vi "SDO_DRIVE_MODULE_ACT.vi"(6 "Pass_Through_Time":dbl=-1.0 format="%33.4f", 8 "AllSwervePosInDeadband":bool=TRUE, 9 "Swerve State":T1={"Speed"=0.0, "Angle"={"VALUE"=0.0, "COS"=1.0, "SIN"=0.0}} {"Angle"."SIN" format="%13.4f"; "Angle"."COS" format="%13.4f"; "Angle"."VALUE" format="%13.4f"}, 10 "Swerve Dmd":T1={"Speed"=0.0, "Angle"={"VALUE"=0.0, "COS"=1.0, "SIN"=0.0}} {"Angle"."SIN" format="%13.4f"; "Angle"."COS" format="%13.4f"; "Angle"."VALUE" format="%13.4f"}, 11 "Swerve Module TypDef":T3) -> (0 "SwerveOnTarget":bool, 1 "SwervePosError":dbl, 2 "Swerve Motor Dmd":dbl, 3 "Wheel Motor Dmd":dbl, 4 "WheelSpeedErr":dbl, 5 "Optimized Swerve \nDmd Radians":dbl, 7 "Optimized Speed \nDmd M/S":dbl)   [LabVIEW 2019]
uses:
  PPS_DRIVE_MODULE_TYPDEF.ctl
  <vilib>/Rock Robotics/WPI/MotorControl/WPI_MotorControlDeviceRef.ctl
  <vilib>/Rock Robotics/WPI/MotorControl/WPI_MotorControlType.ctl
  <vilib>/Rock Robotics/SystemInterfaces/DIO/FPGA_DIOPWMChannel.ctl
  <vilib>/Rock Robotics/WPI/PWM/WPI_PWMDeadband.ctl
  <vilib>/Rock Robotics/SystemInterfaces/DIO/FPGA_DIOChannel.ctl
  <vilib>/Rock Robotics/WPI/Encoder/WPI_EncoderDevRef.ctl
  <vilib>/Rock Robotics/SystemInterfaces/Encoder/FPGA_EncoderIdx.ctl
  <vilib>/Rock Robotics/SystemInterfaces/Counter/FPGA_CounterCtrSystemIndex.ctl
  <vilib>/Rock Robotics/WPI/Encoder/WPI_EncoderType.ctl
  <vilib>/Rock Robotics/WPI/ThirdParty/JAS_Junk/TrajLib/TypeDef/SWERVE_DRIVE_MODULE_STATE.ctl
  <vilib>/Rock Robotics/WPI/ThirdParty/JAS_Junk/TrajLib/TypeDef/ROTATION2D.ctl
  <vilib>/Rock Robotics/WPI/ThirdParty/JAS_Junk/TrajLib/TypeDef/X_Y_PAIR.ctl
  <vilib>/Rock Robotics/WPI/ThirdParty/JAS_Junk/TrajLib/VI/Util_GetTime_U32.vi
  <vilib>/Rock Robotics/WPI/ThirdParty/JAS_Junk/TrajLib/Rotation2d_Minus.vi
  <vilib>/Rock Robotics/WPI/ThirdParty/JAS_Junk/TrajLib/Rotation2d_GetRadians.vi
  <vilib>/Rock Robotics/WPI/ThirdParty/JAS_Junk/TrajLib/SwerveModuleState_New.vi
  <vilib>/Rock Robotics/WPI/ThirdParty/JAS_Junk/TrajLib/Rotation2d_RotateBy.vi
  <vilib>/Rock Robotics/WPI/ThirdParty/JAS_Junk/TrajLib/Rotation2d_CreateAngle.vi
  <vilib>/Rock Robotics/WPI/ThirdParty/JAS_Junk/TrajLib/ProfiledPIDController_SetPID.vi
  <vilib>/Rock Robotics/WPI/ThirdParty/JAS_Junk/TrajLib/ProfiledPIDController_SetIntegratorRange.vi
  <vilib>/Rock Robotics/WPI/ThirdParty/JAS_Junk/TrajLib/ProfiledPIDController_SetTolerance_PosVel.vi
  <vilib>/Rock Robotics/WPI/ThirdParty/JAS_Junk/TrajLib/ProfiledPIDController_DisableContInput.vi
  <vilib>/Rock Robotics/WPI/ThirdParty/JAS_Junk/TrajLib/ProfiledPIDController_EnableContInput.vi
  <vilib>/Rock Robotics/WPI/ThirdParty/JAS_Junk/TrajLib/ProfiledPIDController_Reset_PosOnly.vi
  <vilib>/Rock Robotics/WPI/ThirdParty/JAS_Junk/TrajLib/ProfiledPIDController_NewPeriod.vi
  <vilib>/Rock Robotics/WPI/ThirdParty/JAS_Junk/TrajLib/ProfiledPIDController_Calculate_Meas_Goal.vi
  <vilib>/Rock Robotics/WPI/ThirdParty/JAS_Junk/TrajLib/ProfiledPIDController_AtGoal.vi
  <vilib>/Rock Robotics/WPI/ThirdParty/JAS_Junk/TrajLib/ProfiledPIDController_AtSetpoint.vi
  <vilib>/Rock Robotics/WPI/ThirdParty/JAS_Junk/TrajLib/ProfiledPIDController_SetConstraints.vi
  <vilib>/Rock Robotics/WPI/ThirdParty/JAS_Junk/TrajLib/VI/FunctionGenerator_New.vi
  <vilib>/Rock Robotics/WPI/ThirdParty/JAS_Junk/TrajLib/VI/FunctionGenerator_Calculate.vi
  <vilib>/Rock Robotics/WPI/ThirdParty/JAS_Junk/TrajLib/PIDController_AtSetpoint.vi
  <vilib>/Rock Robotics/WPI/ThirdParty/JAS_Junk/TrajLib/PIDController_SetPIDF.vi
  <vilib>/Rock Robotics/WPI/ThirdParty/JAS_Junk/TrajLib/PIDController_SetDerivativeFilter.vi
  <vilib>/Rock Robotics/WPI/ThirdParty/JAS_Junk/TrajLib/PIDController_SetIntegratorRange.vi
  <vilib>/Rock Robotics/WPI/ThirdParty/JAS_Junk/TrajLib/PIDController_SetTolerancePandV.vi
  <vilib>/Rock Robotics/WPI/ThirdParty/JAS_Junk/TrajLib/PIDController_DisableContinousInput.vi
  <vilib>/Rock Robotics/WPI/ThirdParty/JAS_Junk/TrajLib/PIDController_EnableContinousInput.vi
  <vilib>/Rock Robotics/WPI/ThirdParty/JAS_Junk/TrajLib/PIDController_Reset.vi
  <vilib>/Rock Robotics/WPI/ThirdParty/JAS_Junk/TrajLib/PIDController_New.vi
  <vilib>/Rock Robotics/WPI/ThirdParty/JAS_Junk/TrajLib/PIDController_SetOutputLimits.vi
  <vilib>/Rock Robotics/WPI/ThirdParty/JAS_Junk/TrajLib/SlewRateLimiter_New.vi
  <vilib>/Rock Robotics/WPI/ThirdParty/JAS_Junk/TrajLib/SlewRateLimiter_Reset.vi
  <vilib>/Rock Robotics/WPI/ThirdParty/JAS_Junk/TrajLib/SlewRateLimiter_Calculate.vi
  <vilib>/Rock Robotics/WPI/ThirdParty/JAS_Junk/TrajLib/SlewRateLimiter_SetRate.vi
  <vilib>/Rock Robotics/WPI/ThirdParty/JAS_Junk/TrajLib/Rotation2d_UnaryMinus.vi
  <vilib>/Rock Robotics/WPI/ThirdParty/JAS_Junk/TrajLib/Rotation2d_CreateXY.vi
  <vilib>/Rock Robotics/WPI/ThirdParty/JAS_Junk/TrajLib/PIDController_SetPID.vi
  <vilib>/Rock Robotics/WPI/ThirdParty/JAS_Junk/TrajLib/TrapProfState_New.vi
  <vilib>/Rock Robotics/WPI/ThirdParty/JAS_Junk/TrajLib/ProfiledPIDController_Reset.vi
  <vilib>/Rock Robotics/WPI/ThirdParty/JAS_Junk/TrajLib/PIDController_NewPeriod.vi
  <vilib>/Rock Robotics/SystemInterfaces/NetworkCommunication/NetComm_UsageReport_report.vi
  <vilib>/Rock Robotics/WPI/ThirdParty/JAS_Junk/TrajLib/ProfiledPIDController_SetGoal_PosOnly.vi
  <vilib>/Rock Robotics/WPI/ThirdParty/JAS_Junk/TrajLib/ProfiledPIDController_Calculate_Meas.vi
  <vilib>/Rock Robotics/WPI/ThirdParty/JAS_Junk/TrajLib/TrapProfState_Equals.vi
  <vilib>/Rock Robotics/WPI/ThirdParty/JAS_Junk/TrajLib/Util_CalcDist.vi
  <vilib>/Rock Robotics/WPI/ThirdParty/JAS_Junk/TrajLib/ProfiledPIDController_SetGoal.vi
  <vilib>/Rock Robotics/WPI/ThirdParty/JAS_Junk/TrajLib/PIDController_Calculate_SP_PV.vi
  <vilib>/Rock Robotics/WPI/ThirdParty/JAS_Junk/TrajLib/TrapProfile_New.vi
  <vilib>/Rock Robotics/WPI/ThirdParty/JAS_Junk/TrajLib/ProfiledPIDController_GetPeriod.vi
  <vilib>/Rock Robotics/WPI/ThirdParty/JAS_Junk/TrajLib/TrapProfile_Calculate.vi
  <vilib>/Rock Robotics/WPI/ThirdParty/JAS_Junk/TrajLib/ControllerUtil_GetModulusError.vi
  <vilib>/Rock Robotics/WPI/ThirdParty/JAS_Junk/TrajLib/PIDController_SetSetpoint.vi
  <vilib>/Rock Robotics/WPI/ThirdParty/JAS_Junk/TrajLib/PIDController_Calculate_PV.vi
  <vilib>/Rock Robotics/WPI/ThirdParty/JAS_Junk/TrajLib/TrapProfile_ShouldFlipAcceleration.vi
  <vilib>/Rock Robotics/WPI/ThirdParty/JAS_Junk/TrajLib/TrapProfile_Direct.vi
  <vilib>/Rock Robotics/WPI/ThirdParty/JAS_Junk/TrajLib/PIDController_GetPeriod.vi
  <vilib>/Rock Robotics/WPI/ThirdParty/JAS_Junk/TrajLib/VI/Util_GetTime_U64.vi
  <vilib>/gmath/interp.llb/Search Ordered Table.vi
  <vilib>/Rock Robotics/WPI/ThirdParty/JAS_Junk/TrajLib/Globals/Util_LibraryGlobals.vi
  SDO_DRIVE_GLOBALS.vi
  <vilib>/Rock Robotics/WPI/ThirdParty/JAS_Junk/TrajLib/PIDController_AdvCalculate_FF_Sp_Pv.vi
  <vilib>/Rock Robotics/WPI/ThirdParty/JAS_Junk/TrajLib/Trajectory_Library.lvlib
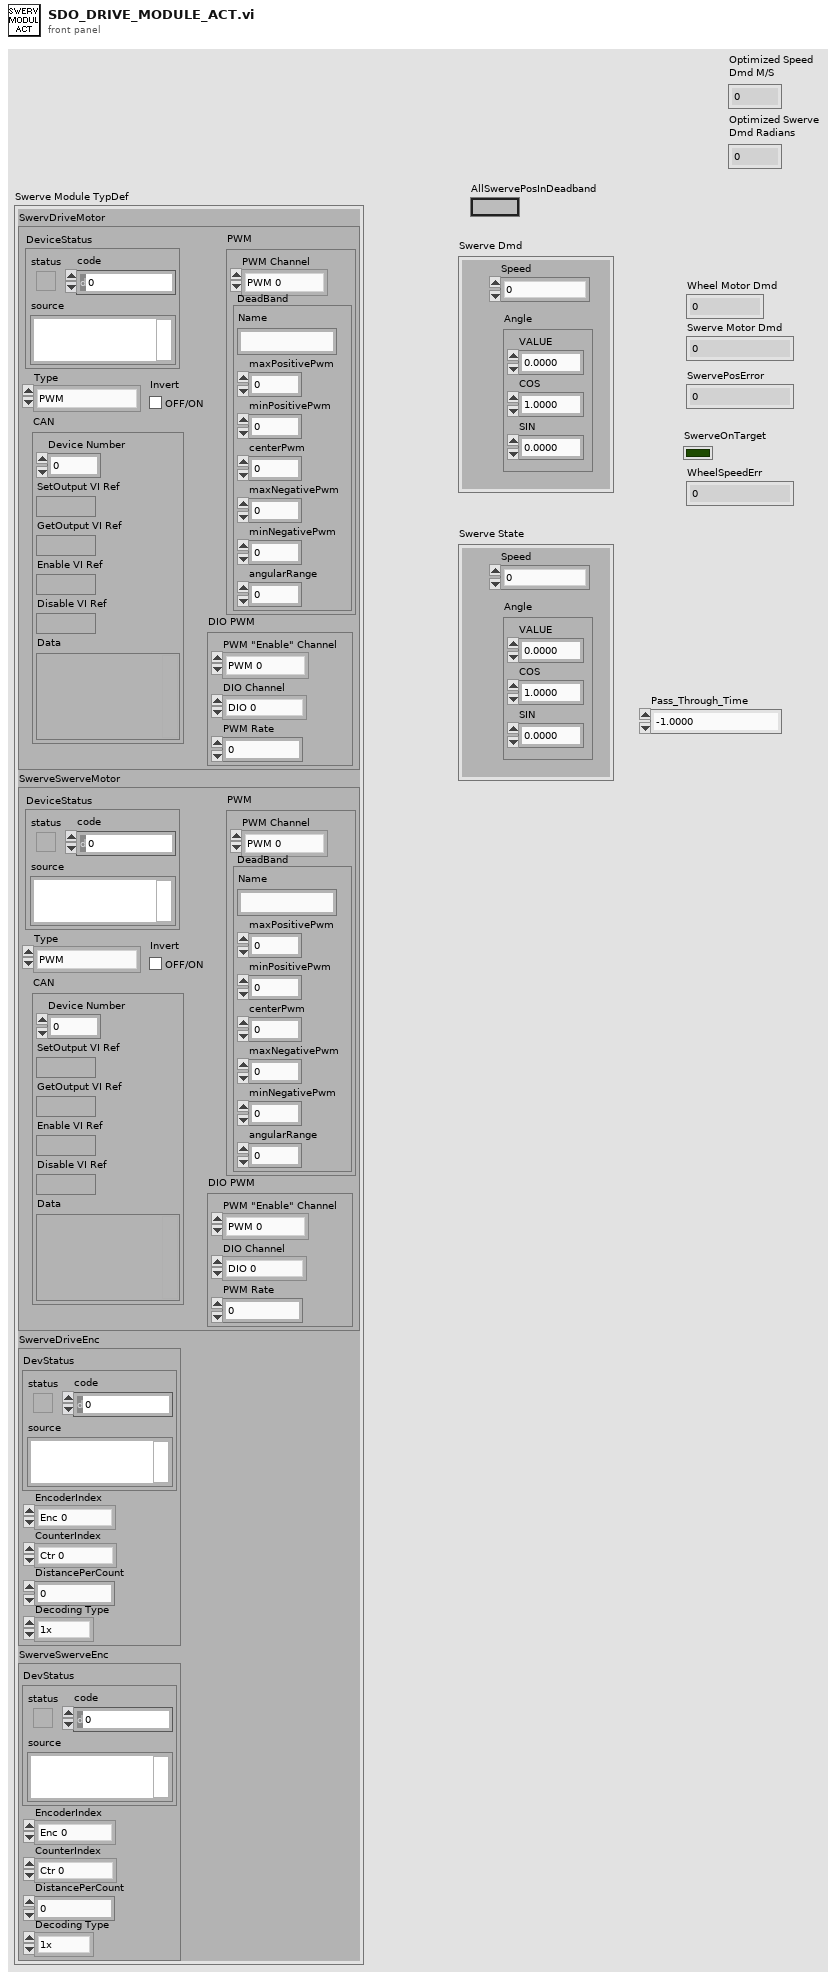
[diagram p1: front panel]
types:
  T1 = typedef "Trajectory_Library.lvlib/SWERVE_DRIVE_MODULE_STATE.ctl" = cluster{"Speed":dbl, "Angle":T2}
  T2 = typedef "Trajectory_Library.lvlib/ROTATION2D.ctl" = cluster{"VALUE":dbl, "COS":dbl, "SIN":dbl}
  T3 = typedef "PPS_DRIVE_MODULE_TYPDEF.ctl" = cluster{"SwervDriveMotor":T4, "SwerveSwerveMotor":T4, "SwerveDriveEnc":T9, "SwerveSwerveEnc":T9}
  T4 = typedef "WPI_MotorControlDeviceRef.ctl" = cluster{"DeviceStatus":errorcluster, "Type":T5, "PWM":cluster{"PWM Channel":T6, "DeadBand":T7}, "CAN":cluster{"Device Number":u8, "SetOutput VI Ref":variant, "GetOutput VI Ref":variant, "Enable VI Ref":variant, "Disable VI Ref":variant, "Data":variant}, "Invert":bool, "DIO PWM":cluster{"PWM \"Enable\" Channel":T6, "DIOChannel":T8, "PWM Rate":dbl}}
  T5 = typedef "WPI_MotorControlType.ctl" = enum16{"PWM", "CAN", "DIO PWM"}
  T6 = typedef "FPGA_DIOPWMChannel.ctl" = enum8{"PWM 0", "PWM 1", "PWM 2", "PWM 3", "PWM 4", "PWM 5", "PWM 6", "PWM 7", "PWM 8", "PWM 9", "PWM MXP 0", "PWM MXP 1", "PWM MXP 2", "PWM MXP 3", "PWM MXP 4", "PWM MXP 5", "PWM MXP 6", "PWM MXP 7", "PWM MXP 8", "PWM MXP 9", "Invalid"}
  T7 = typedef "WPI_PWMDeadband.ctl" = cluster{"Name":string, "maxPositivePwm":i32, "minPositivePwm":i32, "centerPwm":i32, "maxNegativePwm":i32, "minNegativePwm":i32, "angularRange":u16}
  T8 = typedef "FPGA_DIOChannel.ctl" = enum8{"DIO 0", "DIO 1", "DIO 2", "DIO 3", "DIO 4", "DIO 5", "DIO 6", "DIO 7", "DIO 8", "DIO 9", "DIO MXP 0", "DIO MXP 1", "DIO MXP 2", "DIO MXP 3", "DIO MXP 4", "DIO MXP 5", "DIO MXP 6", "DIO MXP 7", "DIO MXP 8", "DIO MXP 9", "DIO MXP 10", "DIO MXP 11", "DIO MXP 12", "DIO MXP 13", "DIO MXP 14", "DIO MXP 15", "SPI Port CS1", "SPI Port CS2", "SPI Port CS3", "SPI Port MISO", "SPI Port MOSI", "Invalid"}
  T9 = typedef "WPI_EncoderDevRef.ctl" = cluster{"DevStatus":errorcluster, "EncoderIndex":T10, "CounterIndex":T11, "DistancePerCount":dbl, "Decoding Type":T12}
  T10 = typedef "FPGA_EncoderIdx.ctl" = enum8{"Enc 0", "Enc 1", "Enc 2", "Enc 3", "Enc 4", "Enc 5", "Enc 6", "Enc 7", "Invalid"}
  T11 = typedef "FPGA_CounterCtrSystemIndex.ctl" = enum8{"Ctr 0", "Ctr 1", "Ctr 2", "Ctr 3", "Ctr 4", "Ctr 5", "Ctr 6", "Ctr 7", "Invalid"}
  T12 = typedef "WPI_EncoderType.ctl" = enum16{"1x", "2x", "4x"}
  T13 = typedef "Trajectory_Library.lvlib/X_Y_PAIR.ctl" = cluster{"X":dbl, "Y":dbl}
  T14 = typedef "Trajectory_Library.lvlib/PID_TUNING.ctl" = cluster{"Kp":dbl, "Ki":dbl, "Kd":dbl, "MaximumIntegral":dbl, "MinimumIntegral":dbl}
  T15 = typedef "Trajectory_Library.lvlib/PID_ERROR_TOLERANCE.ctl" = cluster{"PositionTolerance":dbl, "VelocityTolerance":dbl}
  T16 = typedef "Trajectory_Library.lvlib/PID_INPUT_LIMITS.ctl" = cluster{"MaxInput":dbl, "MinInput":dbl, "Continuous":bool}
  T17 = typedef "Trajectory_Library.lvlib/TRAPEZOID_PROFILE_CONSTRAINT.ctl" = cluster{"MaxVelocity":dbl, "MaxAcceleration":dbl}
  T18 = typedef "Trajectory_Library.lvlib/PosCtrl_Tuning_Type.ctl" = cluster{"Slope":dbl, "Offset":dbl, "Error Deadband":dbl, "At Reference Count":i32, "Negate Output":bool, "Max Allowd Position":dbl, "Min Allowd Position":dbl}
  T19 = typedef "Trajectory_Library.lvlib/PID_ADV_LIMITS.ctl" = cluster{"MaxInput":dbl, "MinInput":dbl, "Continuous":bool, "MaxOutput":dbl, "MinOutput":dbl}
  T20 = typedef "Trajectory_Library.lvlib/PID_ADV_TUNING.ctl" = cluster{"Kf":dbl, "Kp":dbl, "Ki":dbl, "Kd":dbl, "MaximumIntegral":dbl, "MinimumIntegral":dbl, "Filter Derivative":bool}
  T21 = typedef "Trajectory_Library.lvlib/PID_CONTROLLER.ctl" = cluster{"Kp":dbl, "Ki":dbl, "Kd":dbl, "Period":dbl, "Max_Integral":dbl, "Min_Integral":dbl, "Max_Input":dbl, "Min_Input":dbl, "Continuous":bool, "PositionError":dbl, "VelocityError":dbl, "PrevError":dbl, "TotalError":dbl, "PositionTolerance":dbl, "VelocityTolerance":dbl, "SetPoint":dbl, "Kf":dbl, "Prev_Deriv":dbl, "Prev_Deriv 2":dbl, "DerivativeFilter":bool, "Min_Output":dbl, "Max_Output":dbl, "Prev_F_P":dbl, "Prev_F_P_2":dbl, "AntiWindupActive":bool, "Measurement":dbl}
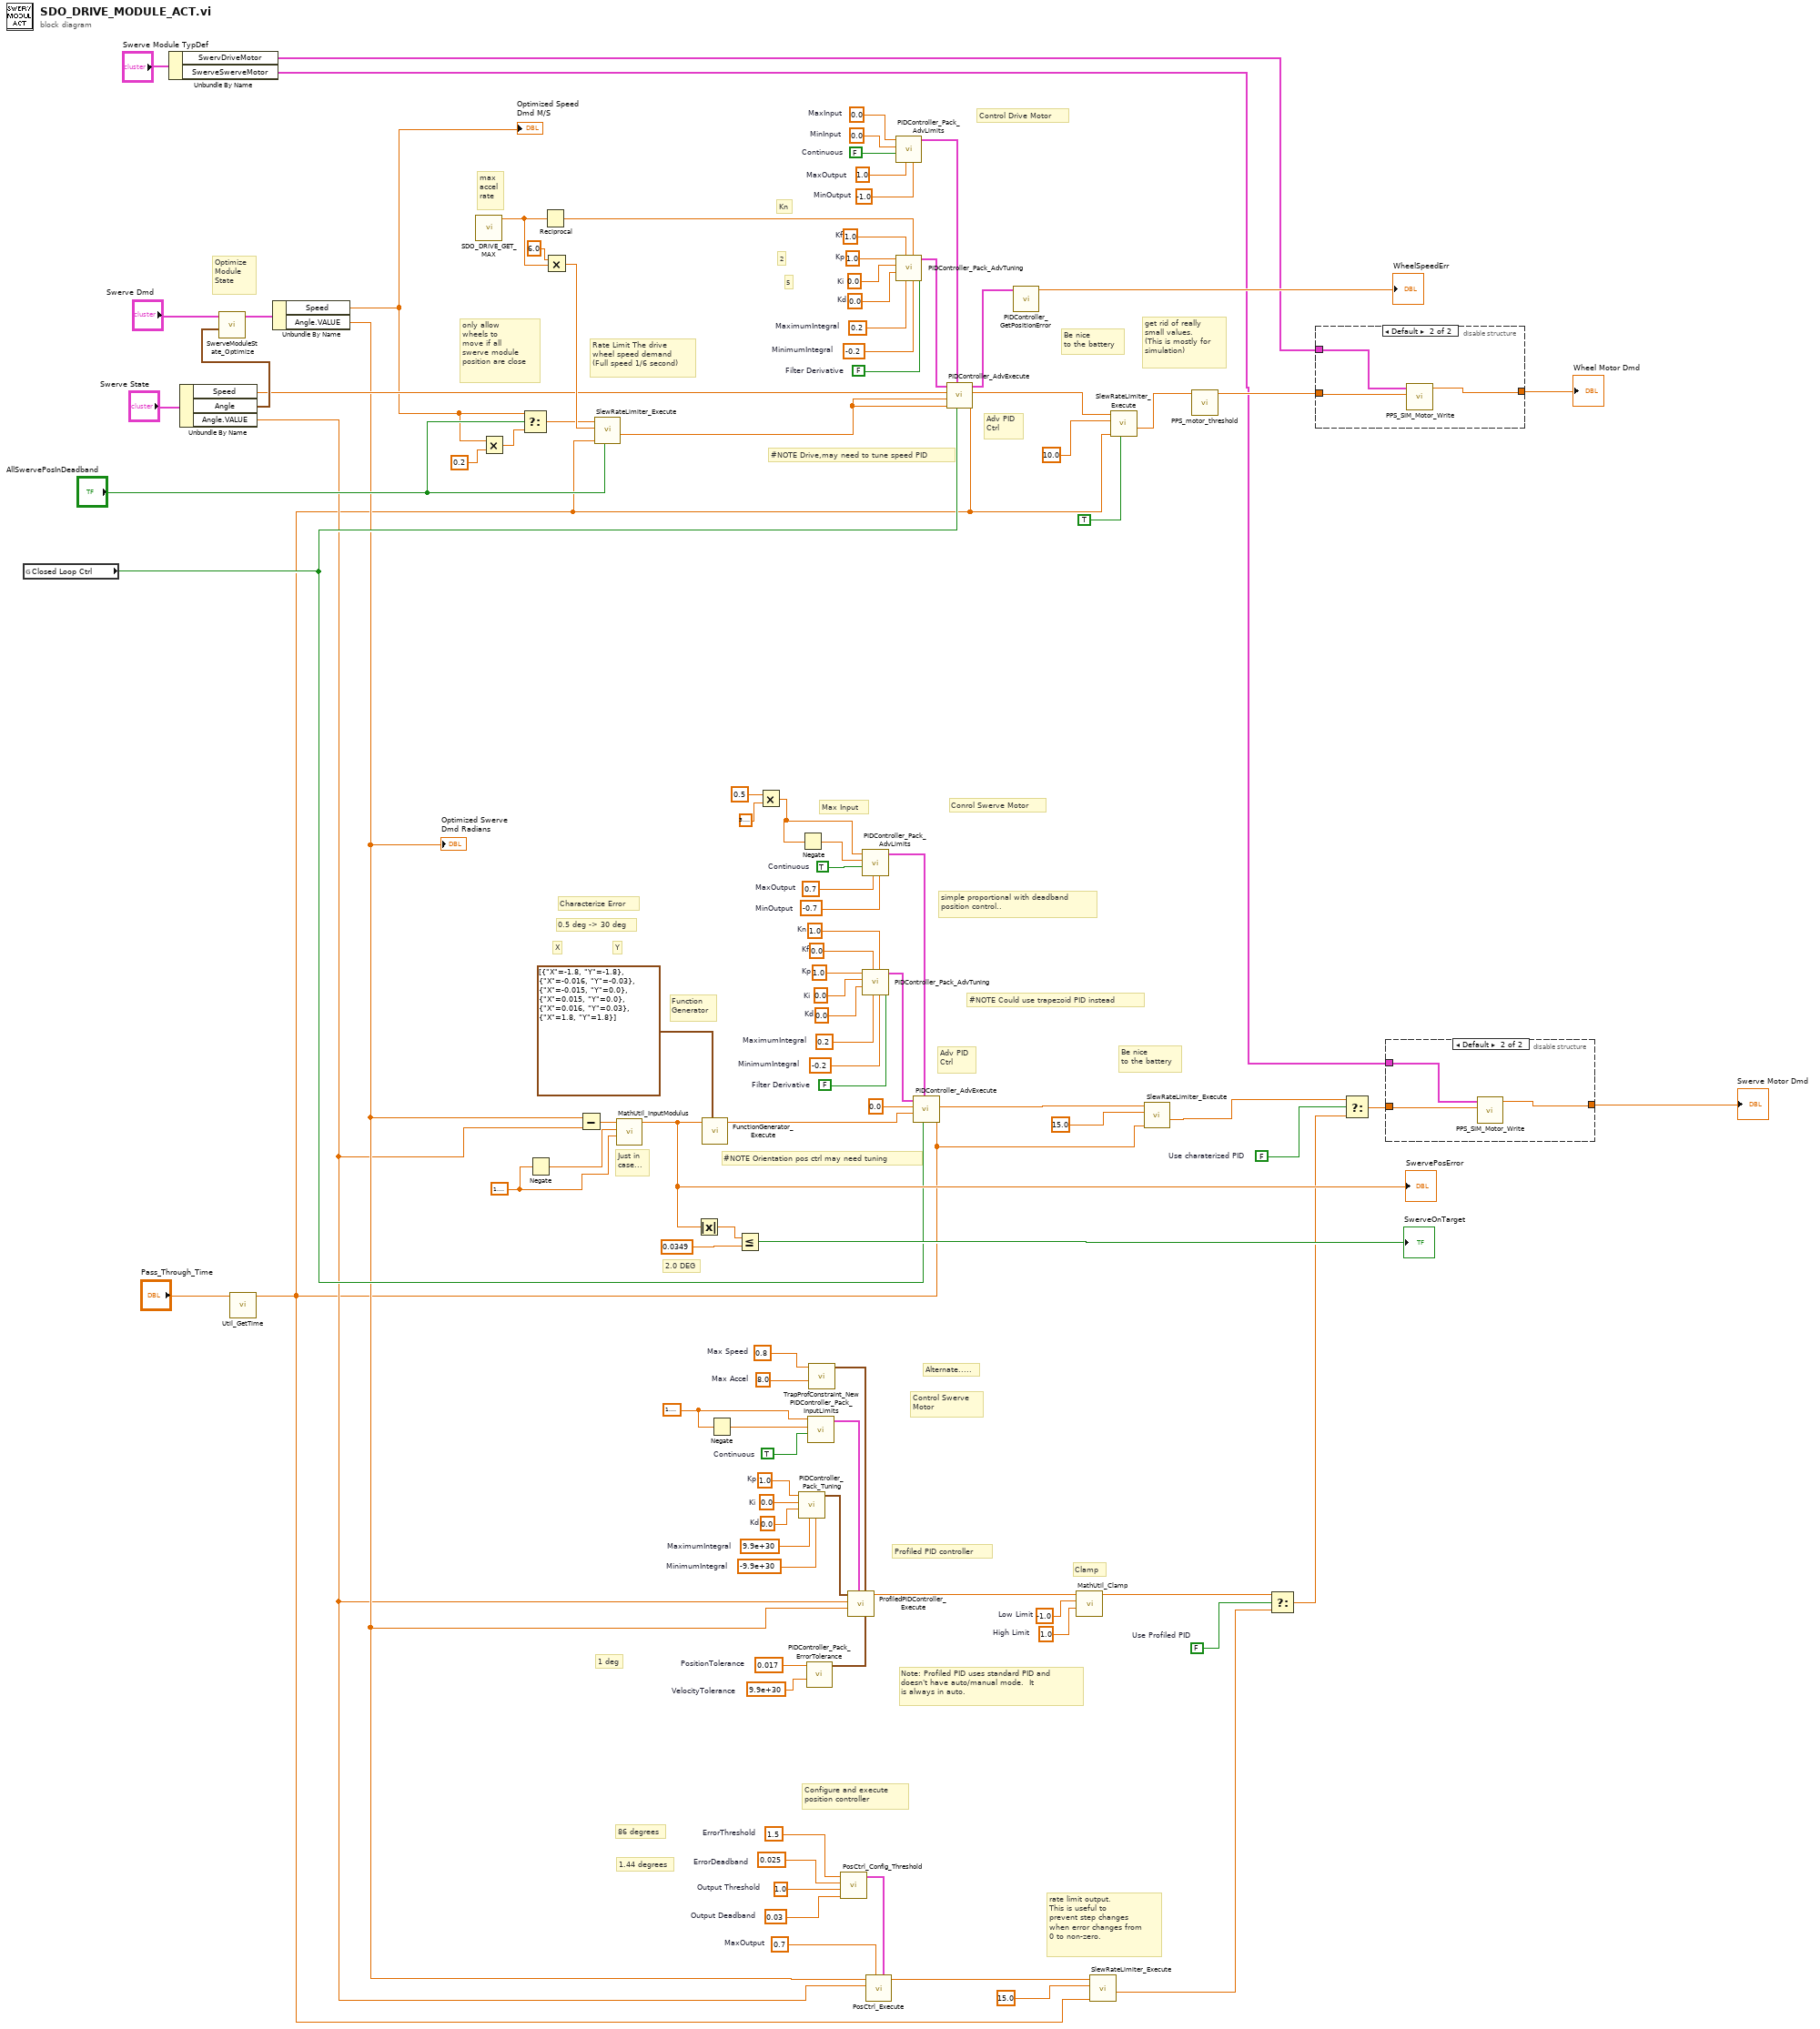
[diagram p0: block diagram]
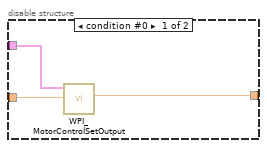
[diagram p2: hidden frame]
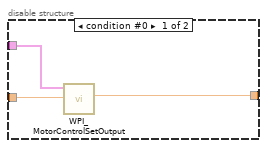
[diagram p3: hidden frame]
diagram:
  w3 = FALSE  # Use charaterized PID
  w11 = FALSE  # Use Profiled PID
  w18 = 0.7  # MaxOutput
  w16 = 1.5  # ErrorThreshold
  w15 = 0.025  # ErrorDeadband
  w14 = 1.0  # Output Threshold
  w13 = 0.03  # Output Deadband
  w22 = 1.5707963267948966
  w23 = 1.5707963267948966
  w29 = 1.0  # High Limit
  w28 = -1.0  # Low Limit
  w54 = 0.017  # PositionTolerance
  w53 = 9.9e+30  # VelocityTolerance
  w51 = 0.8  # Max Speed
  w50 = 8.0  # Max Accel
  w48 = TRUE  # Continuous
  w47 = 1.0  # Kp
  w46 = 0.0  # Ki
  w45 = 0.0  # Kd
  w44 = 9.9e+30  # MaximumIntegral
  w43 = -9.9e+30  # MinimumIntegral
  w78 = 1.0  # Kp
  w77 = 0.0  # Ki
  w76 = 0.0  # Kd
  w75 = 1.0  # Kf
  w74 = 0.2  # MaximumIntegral
  w73 = -0.2  # MinimumIntegral
  w72 = FALSE  # Filter Derivative
  w70 = 0.0  # MinInput
  w69 = FALSE  # Continuous
  w68 = 1.0  # MaxOutput
  w71 = -1.0  # MinOutput
  w67 = 0.0  # MaxInput
  w87 = 0.7  # MaxOutput
  w88 = -0.7  # MinOutput
  w102 = 1.0  # Kn
  w101 = 1.0  # Kp
  w100 = 0.0  # Ki
  w99 = 0.0  # Kd
  w98 = 0.0  # Kf
  w97 = 0.2  # MaximumIntegral
  w96 = -0.2  # MinimumIntegral
  w95 = FALSE  # Filter Derivative
  w94 = TRUE  # Continuous
  # "1.44 degrees"
  # "rate limit output.\nThis is useful to \nprevent step changes\nwhen error changes from\n0 to non-zero."
  # "86 degrees"
  # "Configure and execute \nposition controller"
  # "Alternate....."
  # "Conrol Swerve Motor"
  # "Note: Profiled PID uses standard PID and \ndoesn't have auto/manual mode.  It\nis always in auto."
  # "Be nice\nto the battery"
  # "2.0 DEG"
  # "Control Drive Motor"
  # "Control Swerve \nMotor"
  # "1 deg"
  # "Clamp"
  # "Be nice\nto the battery"
  # "5"
  # "2"
  # "Profiled PID controller"
  # "Optimize\nModule\nState"
  # "Kn"
  # "Adv PID\nCtrl"
  # "Rate Limit The drive\nwheel speed demand\n(Full speed 1/6 second)"
  # "Just in \ncase..."
  # "#NOTE Could use trapezoid PID instead"
  # "Characterize Error"
  # "Max Input"
  # "Adv PID\nCtrl"
  # "0.5 deg -> 30 deg"
  # "Function\nGenerator"
  # "Y"
  # "X"
  # "#NOTE Orientation pos ctrl may need tuning"
  # "only allow\nwheels to \nmove if all \nswerve module \nposition are close"
  # "#NOTE Drive,may need to tune speed PID"
  # "simple proportional with deadband\nposition control.."
  # "get rid of really\nsmall values.\n(This is mostly for \nsimulation)"
  # "max\naccel\nrate"
  n1 = global read "SDO_DRIVE_GLOBALS.vi" "Closed Loop Ctrl"() -> (w19:bool)
  n2 = Unbundle By Name("Swerve Module TypDef") -> ("SwervDriveMotor"=w59:T4, "SwerveSwerveMotor"=w57:T4)
  n3 = Unbundle By Name("Swerve State") -> ("Speed"=w63:dbl, "Angle"=w81:T2, "Angle.VALUE"=w9:dbl)
  n4 = call <vilib>:"SwerveModuleState_Optimize.vi"("CurrentAngle"=w81, "Desired State"="Swerve Dmd") -> ("out SWERVE_DRIVE_MODULE_STATE"=w80:T1)  [unwired: 9 in]
  n5 = call <vilib>:"Util_GetTime.vi"("Pass_Through_Time"="Pass_Through_Time") -> ("FPGA_Time_Seconds"=w1:dbl)  [unwired: 8 in, 2 out]
  n6 = Unbundle By Name(w80) -> ("Speed"=w35:dbl, "Angle.VALUE"=w10:dbl)
  "Optimized Speed \nDmd M/S" <- w35
  "Optimized Swerve \nDmd Radians" <- w10
  n7 = call "SDO_DRIVE_GET_MAX.vi"() -> ("Max Wheel Vel (Meter/Sec)"=w107:dbl)  [unwired: 10 in, 1 out]
  n8 = Multiply(x=w35, y=0.2) -> (x*y=w33:dbl)
  n9 = Select(t=w35, s="AllSwervePosInDeadband", f=w33) -> (s? t:f=w104:dbl)
  n10 = Negate(x=w23) -> (-x=w24:dbl)
  n11 = Reciprocal(x=w107) -> (1/x=w64:dbl)
  n12 = Multiply(x=6.0, y=w107) -> (x*y=w105:dbl)
  n13 = Subtract(x=w10, y=w9) -> (x-y=w26:dbl)
  n14 = call <vilib>:"SlewRateLimiter_Execute.vi"("Enable"="AllSwervePosInDeadband", "Time"=w1, "PositiveRate"=w105, "Input"=w104) -> ("Output"=w60:dbl)  [unwired: 6 in, 1 out]
  n15 = call <vilib>:"MathUtil_InputModulus.vi"("Maximum_Input"=w23, "Minimum_Input"=w24, "Input"=w26) -> ("modulus"=w25:dbl)  [unwired: 8 in]
  "SwervePosError" <- w25
  n16 = Absolute Value(x=w25) -> (abs(x)=w86:dbl)
  n17 = call <vilib>:"FunctionGenerator_Execute.vi"("X Y Pairs"=T13[] [{"X"=-1.8, "Y"=-1.8}, {"X"=-0.016, "Y"=-0.03}, {"X"=-0.015, "Y"=0.0}, {"X"=0.015, "Y"=0.0}, {"X"=0.016, "Y"=0.03}, {"X"=1.8, "Y"=1.8}], "Input Value"=w25) -> ("Output Value"=w89:dbl)  [unwired: 9 in]
  n18 = Negate(x=w22) -> (-x=w40:dbl)
  n19 = Less Or Equal?(x=w86, y=0.0349 ("ErrDeadband")) -> (x <= y?=→"SwerveOnTarget":bool)
  n20 = Multiply(x=0.5, y=3.141592653589793) -> (x*y=w32:dbl)
  n21 = call <vilib>:"PIDController_Pack_Tuning.vi"("MinimumIntegral"=w43, "MaximumIntegral"=w44, "Kd"=w45, "Ki"=w46, "Kp"=w47) -> ("PID Tuning"=w42:T14)  [unwired: 6 in]
  n22 = Negate(x=w32) -> (-x=w91:dbl)
  n23 = call <vilib>:"PIDController_Pack_ErrorTolerance.vi"("VelocityTolerance"=w53, "PositionTolerance"=w54) -> ("PID Error Tolerance"=w52:T15)  [unwired: 9 in]
  n24 = call <vilib>:"PIDController_Pack_InputLimits.vi"("Continuous"=w48, "MinInput"=w40, "MaxInput"=w22) -> ("PID Input Limits"=w41:T16)  [unwired: 8 in]
  n25 = call <vilib>:"TrapProfConstraint_New.vi"("Max Accel"=w50, "Max Speed (M/S)"=w51) -> ("TRAPEZOID_PROFILE_CONSTRAINT"=w49:T17)  [unwired: 9 in]
  n26 = call <vilib>:"PosCtrl_Config_Threshold.vi"("Output Deadband"=w13, "Output Threshold"=w14, "ErrorDeadband"=w15, "ErrorThreshold"=w16) -> ("PosCtrl_Config_Params"=w17:T18)  [unwired: 7 in]
  n27 = call <vilib>:"ProfiledPIDController_Execute.vi"("PID Error Tolerance"=w52, "Constraints"=w49, "PID Input Limits"=w41, "SP-SetPoint Goal"=w10, "PV-Measurement"=w9, "PID Tuning"=w42) -> ("CO-ControlOutput"=w27:dbl)  [unwired: 2 in, 3 out]
  n28 = call <vilib>:"PIDController_Pack_AdvLimits.vi"("MinOutput"=w88, "MaxOutput"=w87, "Continuous"=w94, "MinInput"=w91, "MaxInput"=w32) -> ("Adv PID Limits"=w92:T19)  [unwired: 6 in]
  n29 = call <vilib>:"PIDController_Pack_AdvTuning.vi"("Filter Derivative"=w95, "MinimumIntegral"=w96, "Kn"=w102, "MaximumIntegral"=w97, "Kf"=w98, "Kd"=w99, "Ki"=w100, "Kp"=w101) -> ("Adv PID Tuning"=w93:T20)  [unwired: 3 in]
  n30 = call <vilib>:"PosCtrl_Execute.vi"("PosCtrl_Config_Params"=w17, "MaxOutput"=w18, "CurrentPosition"=w9, "TargetPosition"=w10) -> ("Output"=w5:dbl)  [unwired: 5 in, 2 out]
  n31 = call <vilib>:"PIDController_Pack_AdvLimits.vi"("MinOutput"=w71, "MaxOutput"=w68, "Continuous"=w69, "MinInput"=w70, "MaxInput"=w67) -> ("Adv PID Limits"=w65:T19)  [unwired: 6 in]
  n32 = call <vilib>:"PIDController_Pack_AdvTuning.vi"("Filter Derivative"=w72, "MinimumIntegral"=w73, "Kn"=w64, "MaximumIntegral"=w74, "Kf"=w75, "Kd"=w76, "Ki"=w77, "Kp"=w78) -> ("Adv PID Tuning"=w66:T20)  [unwired: 3 in]
  n33 = call <vilib>:"PIDController_AdvExecute.vi"("Time"=w1, "Auto"=w19, "Adv PID Limits"=w92, "SP-SetPoint"=w89, "PV-Measurement"=0.0, "Adv PID Tuning"=w93) -> ("CO-ControlOutput"=w20:dbl)  [unwired: 3 in, 2 out]
  n34 = call <vilib>:"PIDController_AdvExecute.vi"("Time"=w1, "Auto"=w19, "Adv PID Limits"=w65, "FF-FeedForward"=w60, "SP-SetPoint"=w60, "PV-Measurement"=w63, "Adv PID Tuning"=w66) -> ("CO-ControlOutput"=w39:dbl, "out PID_CONTROLLER"=w62:T21)  [unwired: 2 in, 1 out]
  n35 = call <vilib>:"PIDController_GetPositionError.vi"("in PID_CONTROLLER"=w62) -> ("PositionError"=→"WheelSpeedErr":dbl)  [unwired: 10 in]
  n36 = call <vilib>:"MathUtil_Clamp.vi"("High Limit"=w29, "Low Limit"=w28, "Value"=w27) -> ("Result"=w12:dbl)  [unwired: 8 in]
  n37 = call <vilib>:"SlewRateLimiter_Execute.vi"("Time"=w1, "PositiveRate"=15.0, "Input"=w5) -> ("Output"=w4:dbl)  [unwired: 7 in, 1 out]
  n38 = call <vilib>:"SlewRateLimiter_Execute.vi"("Enable"=TRUE, "Time"=w1, "PositiveRate"=10.0, "Input"=w39) -> ("Output"=w38:dbl)  [unwired: 6 in, 1 out]
  n39 = call <vilib>:"SlewRateLimiter_Execute.vi"("Time"=w1, "PositiveRate"=15.0, "Input"=w20) -> ("Output"=w7:dbl)  [unwired: 7 in, 1 out]
  n40 = call "PPS_motor_threshold.vi"("motor in"=w38) -> ("motor out"=w58:dbl)  [unwired: 10 in]
  n41 = Select(t=w12, s=w11, f=w4) -> (s? t:f=w8:dbl)
  n42 = disable-structure shown="Default" {
    disable-tunnel: w58 -> [w112 w114]
    disable-tunnel: w59 -> [w111 w115]
    disable-tunnel: [w110 w113] -> w56
    frame condition #0 {
      n43 = call <vilib>:"WPI_MotorControlSetOutput.vi"("Output"=w112, "MotorControlDevRef"=w111) -> ("Motor Output"=w110:dbl)  [unwired: 7 in, 2 out]
    }
    frame condition #1 (active) {
      n44 = call "PPS_SIM_Motor_Write.vi"("Motor Demand"=w114, "Motor Device Reference"=w115) -> ("Out Motor Demand"=w113:dbl)  [unwired: 9 in]
    }
  }
  "Wheel Motor Dmd" <- w56
  n45 = Select(t=w7, s=w3, f=w8) -> (s? t:f=w2:dbl)
  n46 = disable-structure shown="Default" {
    disable-tunnel: w2 -> [w118 w120]
    disable-tunnel: w57 -> [w117 w121]
    disable-tunnel: [w116 w119] -> w55
    frame condition #0 {
      n47 = call <vilib>:"WPI_MotorControlSetOutput.vi"("Output"=w118, "MotorControlDevRef"=w117) -> ("Motor Output"=w116:dbl)  [unwired: 7 in, 2 out]
    }
    frame condition #1 (active) {
      n48 = call "PPS_SIM_Motor_Write.vi"("Motor Demand"=w120, "Motor Device Reference"=w121) -> ("Out Motor Demand"=w119:dbl)  [unwired: 9 in]
    }
  }
  "Swerve Motor Dmd" <- w55
